vi "Initialize.vi"(8 "error in (no error)":errorcluster, 9 "ID Query (T: Check)":bool=TRUE, 10 "Reset (T: Reset)":bool=TRUE, 11 "Yokogawa WT500 in":refnum<class "Yokogawa WT500.lvclass">) -> (0 "error out":errorcluster, 2 "VISA resource name":refnum<visa-resource-name>, 3 "Yokogawa WT500 out":refnum<class "Yokogawa WT500.lvclass">)   [LabVIEW 2016, in "Generic Power Analyzer.lvlib" / "Yokogawa WT500.lvlib" / "Yokogawa WT500.lvclass"]
uses:
  Yokogawa WT500.lvclass
  <instrlib>/ykwt500/ykwt500.llb/YKWT500 Read Numeric (Normal).vi
  Generic Power Analyzer/Generic Power Analyzer.lvclass
panel:
  out "Array 3":i32[](array[numeric])
  out "Array 2":string[](array[string])
  out "Element (1: Element 1)":u16
  out "Numeric Control":i32
  out "Array":i32[](array[numeric])
  out "Actual output":u16[][][](array[numeric])
  out "Element (0: All)":u16
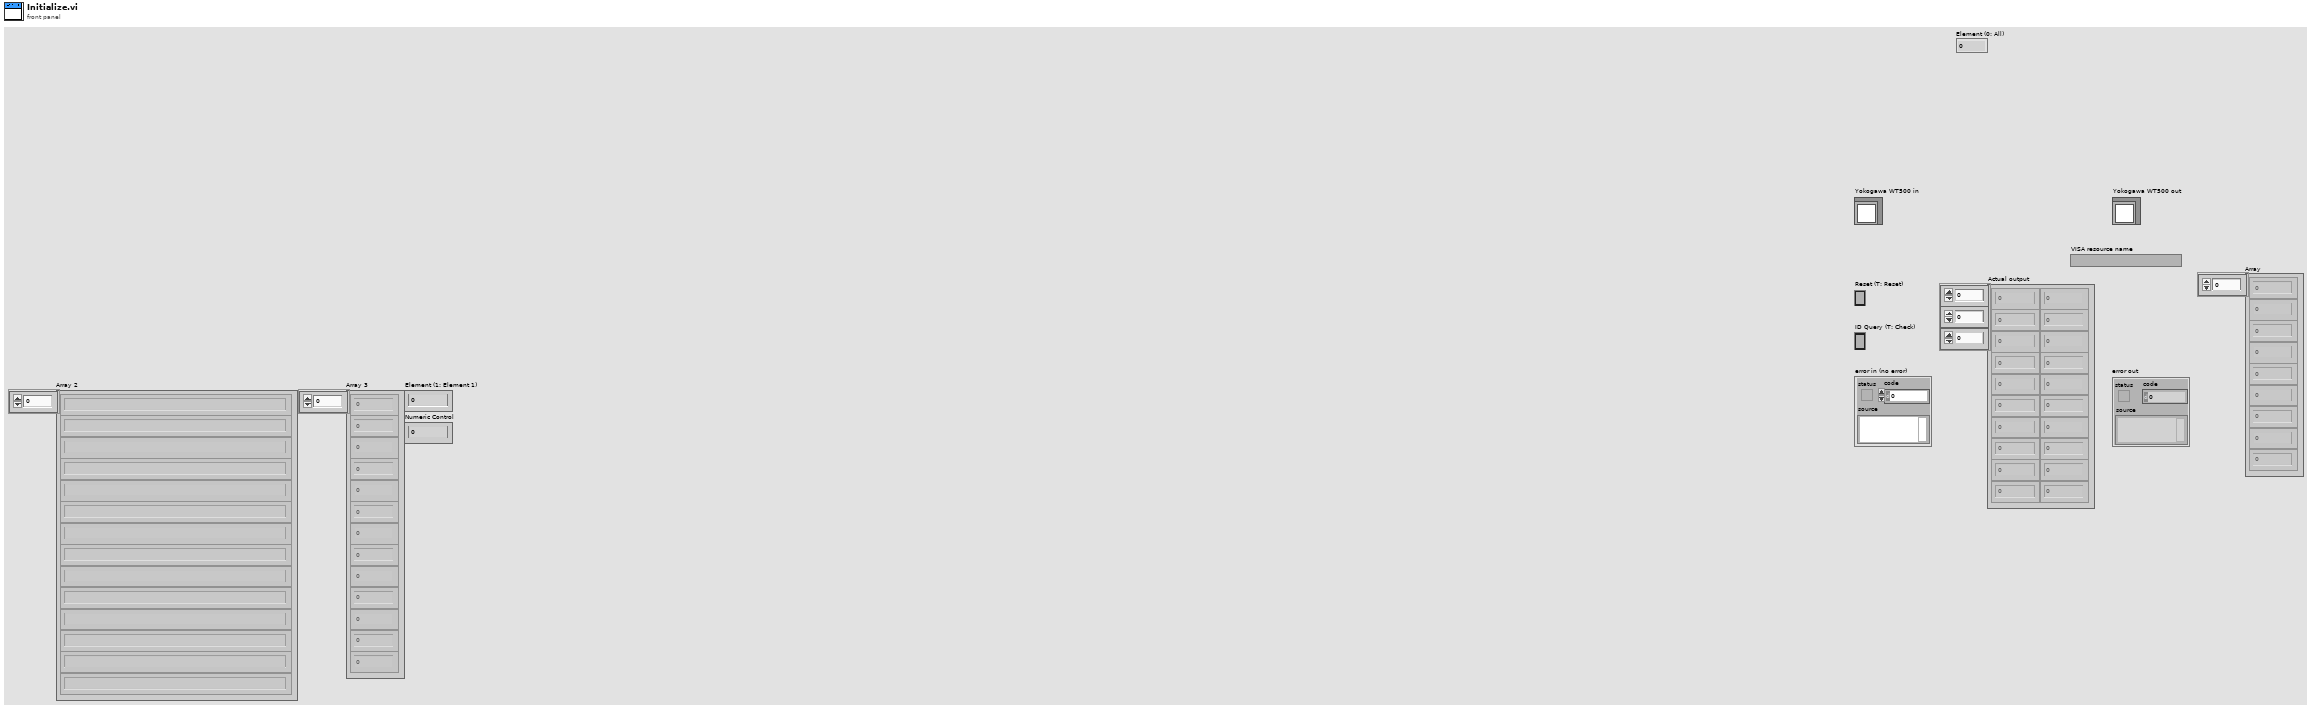
[diagram p1: front panel]
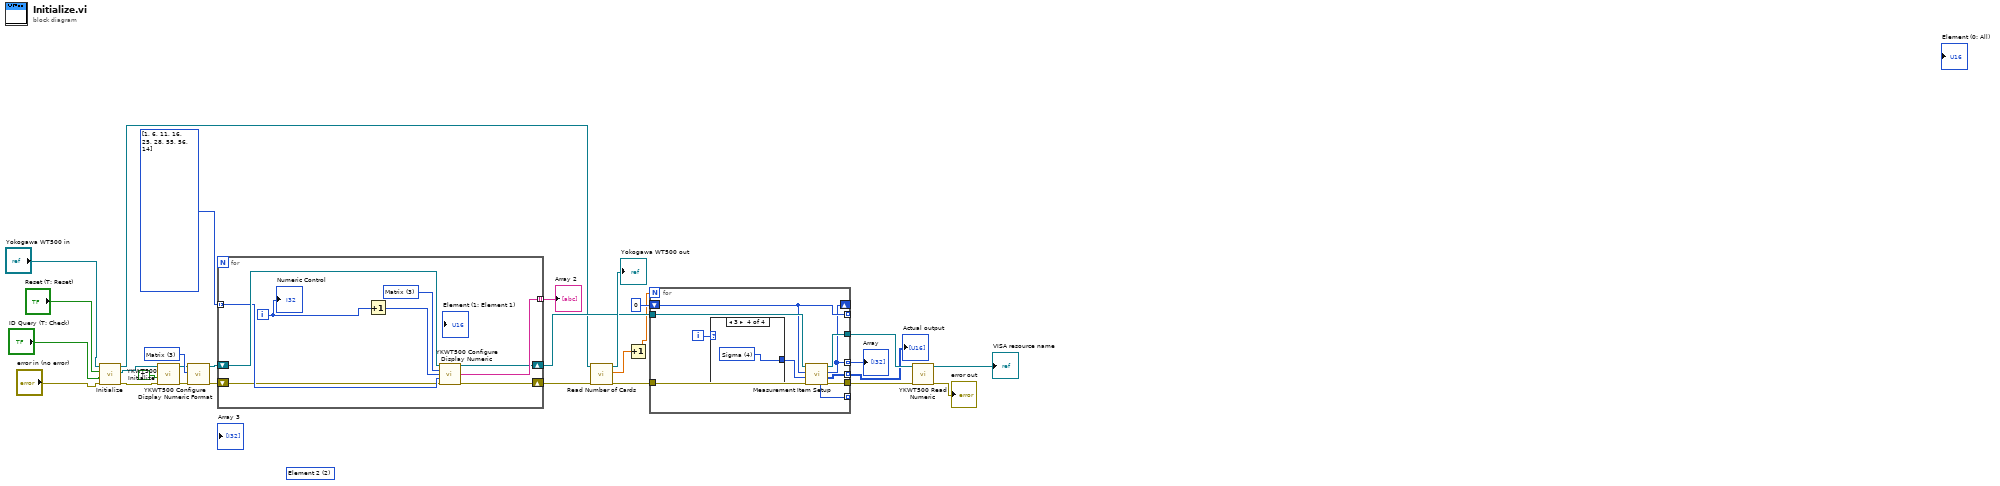
[diagram p0: block diagram]
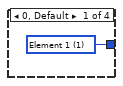
[diagram p2: hidden frame]
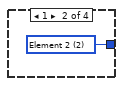
[diagram p3: hidden frame]
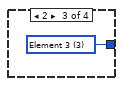
[diagram p4: hidden frame]
diagram:
  (unwired) u16 2 items=["NONE", "Element 1", "Element 2", "Element 3", "Sigma"] ("Element (1: Element 1)")
  w15 = u16[] [1, 6, 11, 16, 25, 28, 55, 56, 14] items=["None", "Urms", "Umn", "Udc", "Urmn", "Uac", "Irms", "Imn", "Idc", "Irmn", "Iac", "P", "S", "Q", "Lambda", "Phi", "Freq U", "Freq I", "U +peak", "U -peak", "I +peak", "I -peak", "Cf U", "Cf I", "Time", "Wp", "Wp+", "Wp-", "q", "q+", "q-", "WS", "WQ", "Eta 1", "Eta 2", "F1", "F2", "F3", "F4", "F5", "F6", "F7", "F8", "U(k)", "I(k)", "P(k)", "S(k)", "Q(k)", "Lambda(k)", "Phi(k)", "Phi U(k)", "Phi I(k)", "Uhdf(k)", "Ihdf(k)", "Phdf(k)", "Uthd", "Ithd", "Pthd", "Phi Ui-Uj", "Phi Ui-Uk", "Phi Ui-Ii", "Phi Ui-Ij", "Phi Ui-Ik", "Delta 1", "Delta 2", "Delta 3", "Delta 4"]
  w18 = u16 3 items=["4 Items", "8 Items", "16 Items", "Matrix", "All", "Single", "Dual"] ("Numeric Format (0: 4 Items)")
  n1 = call-parent "Initialize.vi"("error in (no error)"="error in (no error)", "ID Query"="ID Query (T: Check)", "Reset"="Reset (T: Reset)", "Generic Power Analyzer in"="Yokogawa WT500 in") -> ("error out"=w6:errorcluster, "VISA resource name"=w1:refnum<visa-resource-name>, "Generic Power Analyzer out"=w7:refnum<class "Yokogawa WT500.lvclass">)  [unwired: 5 in]
  n2 = call <instrlib>:"YKWT500 Initialize.vi"("error in (no error)"=w6, "Reset (True)"=TRUE, "VISA resource name"=w1) -> ("error out"=w14:errorcluster, "VISA resource name out"=w11:refnum<visa-resource-name>)  [unwired: 7 in]
  n3 = call <instrlib>:"YKWT500 Configure Display Numeric Format.vi"("error in (no error)"=w14, "Numeric Format (0: 4 Items)"=w18, "VISA resource name"=w11) -> ("error out"=w13:errorcluster, "VISA resource name out"=w17:refnum<visa-resource-name>)  [unwired: 7 in]
  n4 = for {
    tunnel: w15 -> [w35] mode=indexing
    tunnel: [w33] -> w16 mode=indexing
    shift-right: [w30] -> w12
    shift-left: w13 -> [w31]
    shift-right: [w29] -> w10
    shift-left: w17 -> [w37]
    i -> [w32]
    w36 = u16 3 items=["4 Items", "8 Items", "16 Items", "Matrix"] ("Numeric Format (0: 4 Items)")
    n5 = Increment(x=w32) -> (x+1=w34:i32)
    n6 = call <instrlib>:"YKWT500 Configure Display Numeric.vi"("VISA resource name"=w37, "Numeric Format (0: 4 Items)"=w36, "Numeric Item Number (1)"=w34, "Numeric Function (0: None)"=w35, "error in (no error)"=w31) -> ("VISA resource name out"=w29:refnum<visa-resource-name>, "output string"=w33:string, "error out"=w30:errorcluster)  [unwired: 8 in]
    "Numeric Control" <- w32
  }
  "Array 2" <- w16
  n7 = call-dynamic "Read Number of Cards.vi"("error in (no error)"=w12, "Generic Instrument in"=w7) -> ("error out"=w28:errorcluster, "Number of Cards"=w9:dbl, "Generic Instrument out"=→"Yokogawa WT500 out":refnum<class "Yokogawa WT500.lvclass">)  [unwired: 7 in]
  n8 = Increment(x=w9) -> (x+1=w8:dbl)
  n9 = for {
    N: w8 -> [_]
    tunnel: w10 -> [w47]
    tunnel: w28 -> [w46]
    tunnel: [w45] -> w27
    tunnel: [w44] -> w25
    tunnel: [w43] -> w21 mode=indexing
    shift-right: [w38] -> _
    shift-left: 0 ("i-j") -> [w39]
    tunnel: [w40] -> _ mode=indexing
    tunnel: [w39] -> _ mode=indexing
    tunnel: [w38] -> w20 mode=indexing
    i -> [w41]
    n10 = case shown="3" w41 {
      tunnel: [w48 w49 w50 w51] -> w42
      frame 0, Default {
        w48 = u16 1 items=["All", "Element 1", "Element 2", "Element 3", "Sigma"] ("Element (0: All)")
      }
      frame 1 {
        w49 = u16 2 items=["All", "Element 1", "Element 2", "Element 3", "Sigma"] ("Element (0: All)")
      }
      frame 2 {
        w50 = u16 3 items=["All", "Element 1", "Element 2", "Element 3", "Sigma"] ("Element (0: All)")
      }
      frame 3 {
        w51 = u16 4 items=["All", "Element 1", "Element 2", "Element 3", "Sigma"] ("Element (0: All)")
      }
    }
    n11 = call "Measurement Item Setup.vi"("error in (no error)"=w46, "Element (0: All)"=w42, "i-j"=w39, "VISA Refnum in"=w47) -> ("error out"=w44:errorcluster, "Actual output"=w43:u16[][], "i-j 2"=w38:i32, "VISA Refnum out"=w45:refnum<visa-resource-name>, "position"=w40:i32[])  [unwired: 3 in]
  }
  "Actual output" <- w21
  "Array" <- w20
  n12 = call-poly <instrlib>:"YKWT500 Read Numeric.vi"("error in (no error)"=w25, "VISA resource name"=w27) -> ("error out"=→"error out":errorcluster, "VISA resource name out"=→"VISA resource name":refnum<visa-resource-name>)  [unwired: 7 in, 1 out]
